vi "Warning Numerics.vi"() -> ()   [LabVIEW 2020]
panel:
  in  "Thermometer":dbl(slide) scale=-30.0..100.0
  out "Status":string
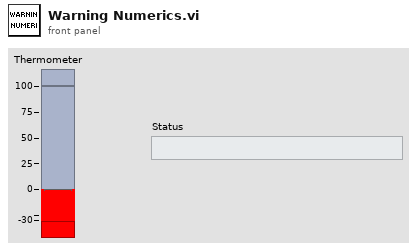
[diagram p1: front panel]
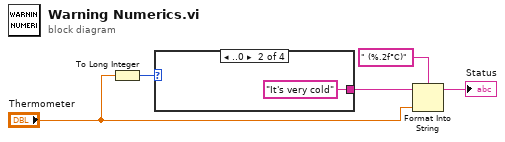
[diagram p0: block diagram]
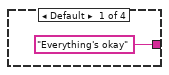
[diagram p2: hidden frame]
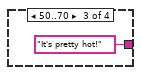
[diagram p3: hidden frame]
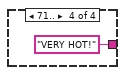
[diagram p4: hidden frame]
diagram:
  n1 = To Long Integer(number="Thermometer") -> (32bit integer=w5:i32)
  n2 = case shown="..0" w5 {
    tunnel: ["Everything's okay" "It's very cold" "It's pretty hot!" "VERY HOT!"] -> w4
    frame Default {
    }
    frame ..0 {
    }
    frame 50..70 {
    }
    frame 71.. {
    }
  }
  n3 = Format Into String(format string=" (%.2f°C)", initial string=w4, "Thermometer") -> (resulting string=→"Status":string)  [unwired: 1 in, 1 out]
